vi "AlliGator Update Local Decay Graph.vi"(8 "Error In":errorcluster, 10 "Profile Window Data":T2[](array[typedef]), 11 "XY Graph Refnum":T1) -> (0 "Error Out":errorcluster)   [LabVIEW 2021, in "AlliGator Local Decay Window.lvlib"]
doc: "Updates the Local Decay Window graph."
uses:
  AlliGator Local Decay Window.lvlib
  Image Profile Window/AlliGator Image Profile Plot Data.ctl
  Graphs/XY Graph/XY Graph Plot Data.ctl
  Graphs/XY Graph/XY Graph Refnum.ctl
  Graphs/XY Graph/XY Graph Add-Ons.lvlib
  Image Profile Window/AlliGator Image Profile Window.lvlib
panel:
  # "see the AlliGator License on the block diagram (Ctrl+E or Window:Show Block Diagram)"
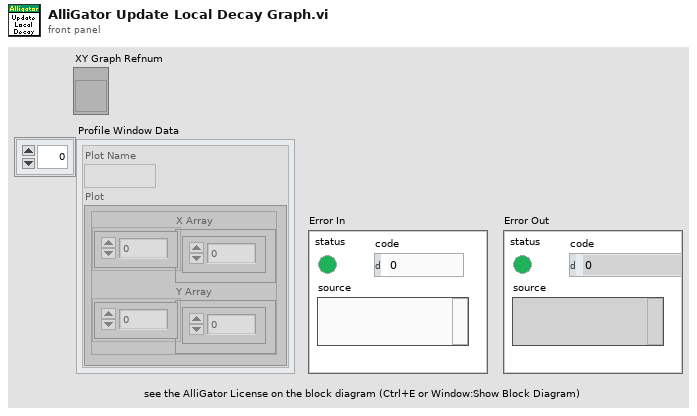
[diagram p1: front panel]
types:
  T1 = typedef "XY Graph Add-Ons.lvlib/XY Graph Refnum.ctl" = refnum<vi>
  T2 = typedef "AlliGator Image Profile Window.lvlib/AlliGator Image Profile Plot Data.ctl" = cluster{"Plot Name":string, "Plot":T3}
  T3 = typedef "XY Graph Add-Ons.lvlib/XY Graph Plot Data.ctl" = cluster{"X Array":dbl[], "Y Array":dbl[]}
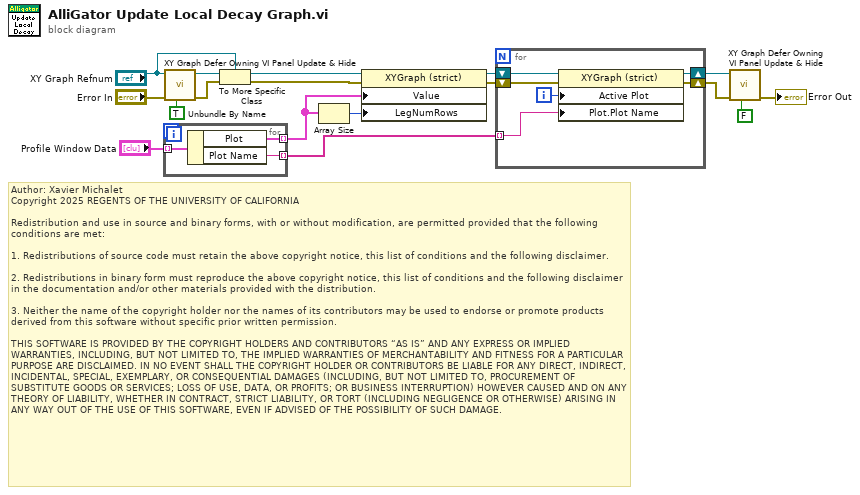
[diagram p0: block diagram]
diagram:
  # "Author: Xavier Michalet\nCopyright 2025 REGENTS OF THE UNIVERSITY OF CALIFORNIA\n\nRedistribution and use in source and binary forms, with or without modification, are permitted provided that the following conditions are met:\n\n1. Redistributions of source code must retain the above copyright notice, this list of conditions and the following disclaimer.\n\n2. Redistributions in binary form must reproduce the above copyright notice, this list of conditions and the following disclaimer in the documentation and/or other materials provided with the distribution.\n\n3. Neither the name of the copyright holder nor the names of its contributors may be used to endorse or promote products derived from this software without specific prior written permission.\n\nTHIS SOFTWARE IS PROVIDED BY THE COPYRIGHT HOLDERS AND CONTRIBUTORS “AS IS” AND ANY EXPRESS OR IMPLIED WARRANTIES, INCLUDING, BUT NOT LIMITED TO, THE IMPLIED WARRANTIES OF MERCHANTABILITY AND FITNESS FOR A PARTICULAR PURPOSE ARE DISCLAIMED. IN NO EVENT SHALL THE COPYRIGHT HOLDER OR CONTRIBUTORS BE LIABLE FOR ANY DIRECT, INDIRECT, INCIDENTAL, SPECIAL, EXEMPLARY, OR CONSEQUENTIAL DAMAGES (INCLUDING, BUT NOT LIMITED TO, PROCUREMENT OF SUBSTITUTE GOODS OR SERVICES; LOSS OF USE, DATA, OR PROFITS; OR BUSINESS INTERRUPTION) HOWEVER CAUSED AND ON ANY THEORY OF LIABILITY, WHETHER IN CONTRACT, STRICT LIABILITY, OR TORT (INCLUDING NEGLIGENCE OR OTHERWISE) ARISING IN ANY WAY OUT OF THE USE OF THIS SOFTWARE, EVEN IF ADVISED OF THE POSSIBILITY OF SUCH DAMAGE."
  n1 = for {
    tunnel: "Profile Window Data" -> [w20] mode=indexing
    tunnel: [w18] -> w6 mode=indexing
    tunnel: [w19] -> w7 mode=indexing
    n2 = Unbundle By Name(w20) -> ("Plot"=w18:T3, "Plot Name"=w19:string)
  }
  n3 = call "XY Graph Defer Owning VI Panel Update & Hide.vi"("Defer Owning Panel Update"=TRUE, "error in (no error)"="Error In", "XY Graph Refnum in"="XY Graph Refnum") -> ("error out"=w11:errorcluster, "XY Graph Refnum out"=w16:refnum<vi>)  [unwired: 7 in]
  n4 = To More Specific Class(target class="XY Graph Refnum", reference=w16, error in=w11) -> (specific class reference=w12:T1, error out=w1:errorcluster)
  n5 = Array Size(array=w6) -> (size(s)=w5:i32)
  n6 = property class="XYGraph (strict)"(reference=w12, error in=w1, "Value"=w6, "LegNumRows"=w5) -> (reference out=w13:T1, error out=w8:errorcluster)
  n7 = for {
    shift-right: [w23] -> w2
    shift-left: w8 -> [w24]
    shift-right: [w25] -> w3
    shift-left: w13 -> [w26]
    tunnel: w7 -> [w21] mode=indexing
    i -> [w22]
    n8 = property class="XYGraph (strict)"(reference=w26, error in=w24, "Active Plot"=w22, "Plot.Plot Name"=w21) -> (reference out=w25:T1, error out=w23:errorcluster)
  }
  n9 = call "XY Graph Defer Owning VI Panel Update & Hide.vi"("Defer Owning Panel Update"=FALSE, "error in (no error)"=w2, "XY Graph Refnum in"=w3) -> ("error out"=→"Error Out":errorcluster)  [unwired: 7 in, 1 out]
